vi "Create Job.vi"(8 "error in (no error)":errorcluster, 10 "Job Name":string, 11 "Job in":refnum<class "Job.lvclass">) -> (0 "error out":errorcluster, 3 "Job":refnum<class "Job.lvclass">)   [LabVIEW 2013, in "openCron.lvlib" / "Job.lvclass"]
uses:
  Job.lvclass
  Job.lvclass/Job.ctl
  Job Report -- cluster.ctl
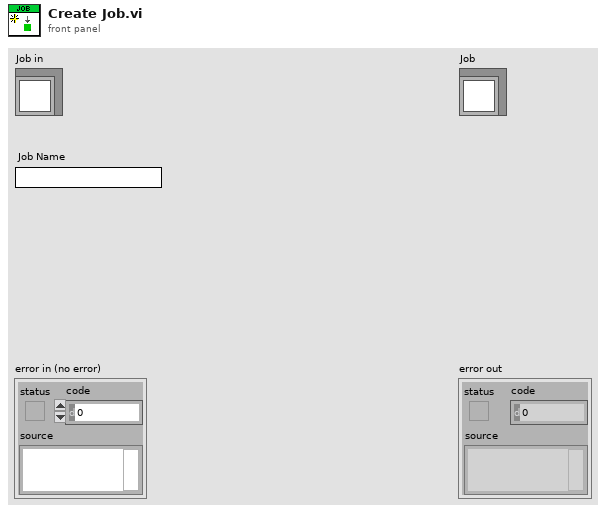
[diagram p1: front panel]
types:
  T1 = typedef "openCron.lvlib/Job.lvclass/Job Report -- cluster.ctl" = cluster{"Name":string, "GUID":string, "Start Time":timestamp, "Duration (s)":dbl, "exception code":i32}
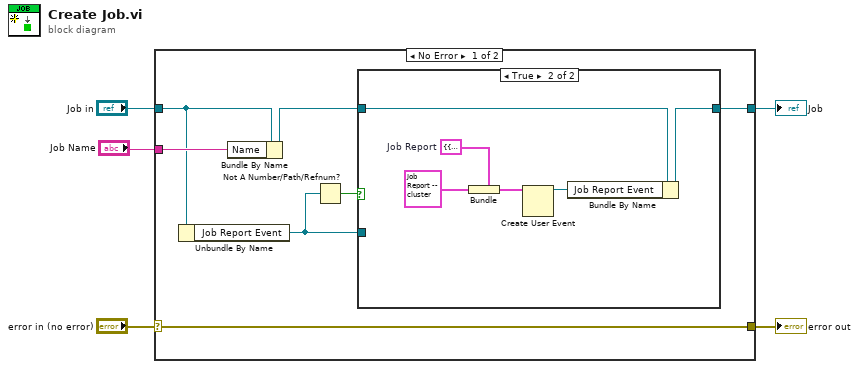
[diagram p0: block diagram]
diagram:
  n1 = case shown="No Error" "error in (no error)" {
    selector: "error in (no error)" -> [w12 w21]
    tunnel: [w12 w21] -> w4
    tunnel: [w11 w20] -> w2
    tunnel: "Job in" -> [w7 w20]
    tunnel: "Job Name" -> [w8 _]
    frame No Error {
      n2 = Unbundle By Name(w7) -> ("Job Report Event"=w9:refnum<user-event>)
      n3 = Bundle By Name(cluster=w7, "Name"=w8) -> (w6:refnum<class "Job.lvclass">)
      n4 = Not A Number/Path/Refnum?(number/path/refnum=w9) -> (NaN/Path/Refnum?=w10:bool)
      n5 = case shown="True" w10 {
        tunnel: [w13 w15] -> w11
        tunnel: w6 -> [w13 w14]
        tunnel: w9 -> [_ _]
        frame False {
          # "Job Report Event already exists"
        }
        frame True {
          w17 = cluster{"Job Report":T1} {"Job Report"={"Name"="", "GUID"="", "Start Time"=timestamp(0 s since 1904-01-01), "Duration (s)"=0.0, "exception code"=0}}  # Job Report
          n6 = Bundle(cluster=w17, "Job Report"=T1 {"Name"="", "GUID"="", "Start Time"=timestamp(0 s since 1904-01-01), "Duration (s)"=0.0, "exception code"=0}) -> (w18:cluster{"Job Report":T1})
          n7 = Create User Event(user event datatype=w18) -> (user event=w16:refnum<user-event>)  [unwired: 1 in, 1 out]
          n8 = Bundle By Name(cluster=w14, "Job Report Event"=w16) -> (w15:refnum<class "Job.lvclass">)
        }
      }
    }
    frame Error {
    }
  }
  "error out" <- w4
  "Job" <- w2
